vi "Test Method Memory.vi"() -> ()   [LabVIEW 2011]
uses:
  Method.ctl
panel:
  out "Method Out":T1
  in  "stop":bool
  in  "ADT version":i32
  in  "Method Name":string
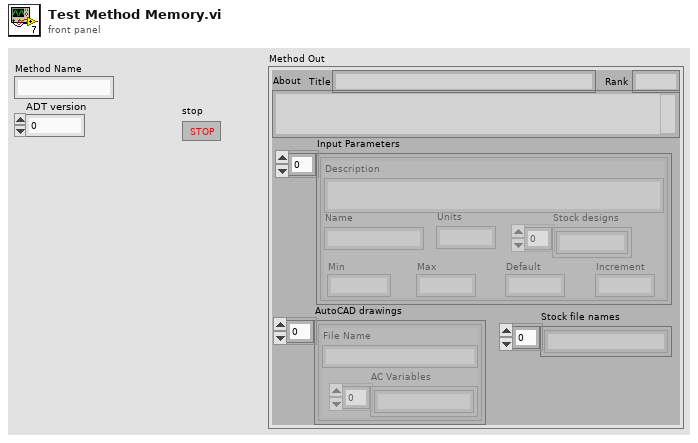
[diagram p1: front panel]
types:
  T1 = typedef "Method.ctl" = cluster{"Title":string, "Rank":string, "About":string, "Input Parameters":cluster{"Description":string, "Name":string, "Min":string, "Max":string, "Default":string, "Units":string, "Increment":string, "Stock designs":string[]}[], "AutoCAD drawings":cluster{"File Name":string, "AC Variables":string[]}[], "Stock file names":string[]}
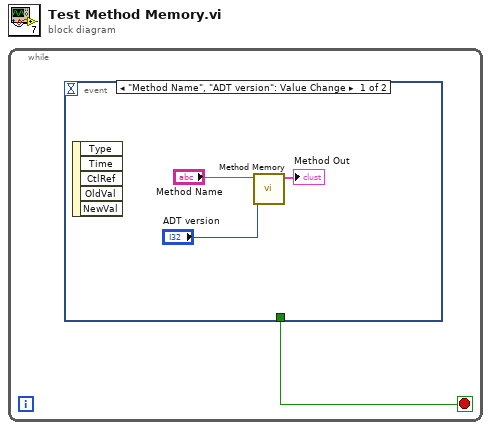
[diagram p0: block diagram]
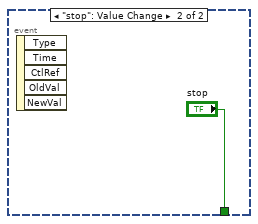
[diagram p2: hidden frame]
diagram:
  n1 = while {
    stop <- w1 stop-if-true
    n2 = event shown="[0] \"Method Name\", \"ADT version\": Value Change" {
      selector: _ -> [_ _]
      dyn-events: _ -> [_ _]
      timeout: _ -> [_ _]
      tunnel: [_ "stop"] -> w1
      event "Method Name", "ADT version": Value Change {
        n3 = event-data() -> ()  [unwired: 1 in, 5 out]
        n4 = call "Method Memory.vi"("ADT version"="ADT version", "Method Name"="Method Name") -> ("Method Out"=→"Method Out":T1)  [unwired: 7 in, 2 out]
      }
      event "stop": Value Change {
        n5 = event-data() -> ()  [unwired: 1 in, 5 out]
      }
    }
  }
